vi "Yokogawa Control.vi"(8 "error in (no error)":errorcluster, 9 "Metadata All":T1={"Data Fields"={"operatorName"="", "project"="", "measurementType"="", "sphere"="", "spectrometer"="", "powerSource"="", "analyzer"="", "fixtureType"="", "lampType"="", "sourceType"="", "testOrientation"="", "model"="", "sample"="", "hours"="", "Amp Gain Range"=""}, "Metadata Disable"={"spectrometer"=enum."Disabled and Grayed Out", "sphere"=enum."Disabled and Grayed Out", "analyzer"=enum."Disabled and Grayed Out", "ampGainRange"=enum."Disabled and Grayed Out"}, "Output Path"=path "C:/Users/dhstuart/Dropbox/CLTC/YokogawaPZ4000/Output"}, 10 "Master":refnum<queue>, 11 "VI in":refnum<vi>) -> (0 "error out":errorcluster, 2 "Electrical Data 2":T4)   [LabVIEW 2013]
uses:
  MeasurementControl Message Queue Folder/Message Cluster.ctl
  YokogawaPZ4000/controls/electrical2.ctl
  controls/Metadata all typedef.ctl
  controls/Metadata typedef.ctl
  controls/Metadata disable typedef.ctl
  YokogawaPZ4000/Acquisition/YKPZ400 Acquisition.lvlib
  MeasurementControl Message Queue Folder/MeasurementControl Message Queue.lvlib
  controls/Metadata.lvlib
panel:
  in  "Boolean":bool
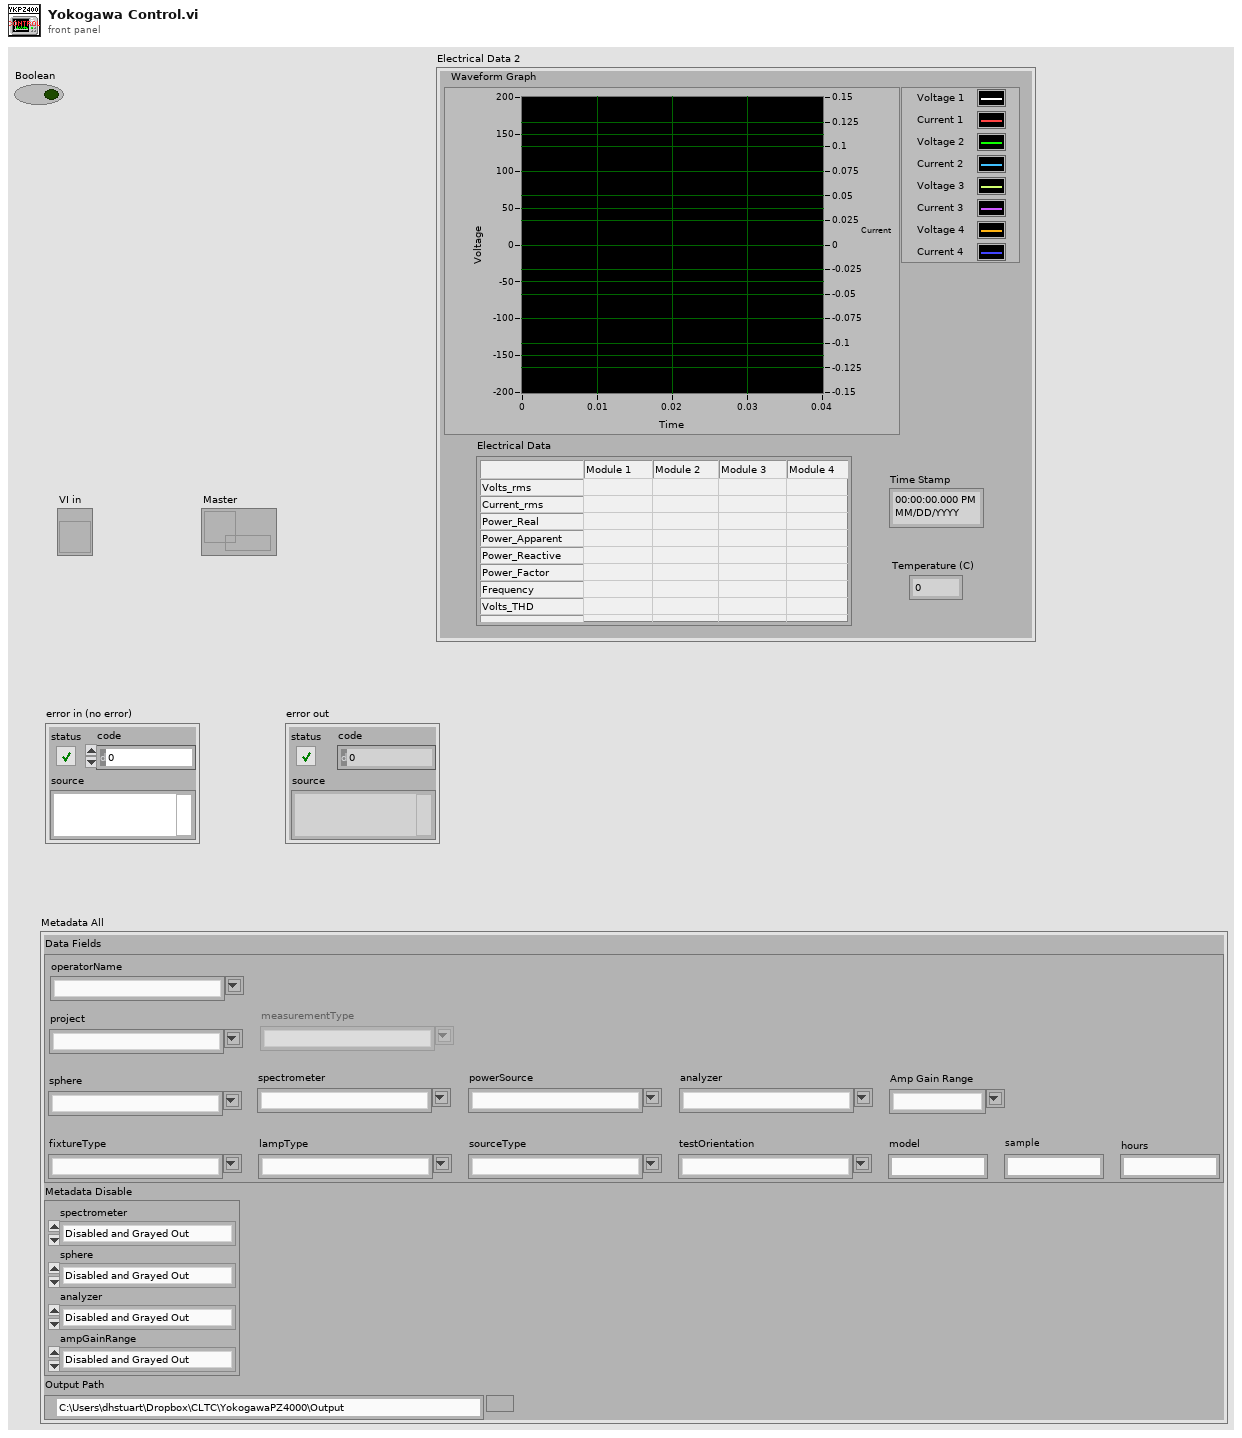
[diagram p1: front panel]
types:
  T1 = typedef "Metadata.lvlib/Metadata all typedef.ctl" = cluster{"Data Fields":T2, "Metadata Disable":T3, "Output Path":path}
  T2 = typedef "Metadata.lvlib/Metadata typedef.ctl" = cluster{"operatorName":string, "project":string, "measurementType":string, "sphere":string, "spectrometer":string, "powerSource":string, "analyzer":string, "fixtureType":string, "lampType":string, "sourceType":string, "testOrientation":string, "model":string, "sample":string, "hours":string, "Amp Gain Range":string}
  T3 = typedef "Metadata.lvlib/Metadata disable typedef.ctl" = cluster{"spectrometer":enum8{"Enabled", "Disabled", "Disabled and Grayed Out"}, "sphere":enum8{"Enabled", "Disabled", "Disabled and Grayed Out"}, "analyzer":enum8{"Enabled", "Disabled", "Disabled and Grayed Out"}, "ampGainRange":enum8{"Enabled", "Disabled", "Disabled and Grayed Out"}}
  T4 = typedef "Yokogawa.lvlib/YKPZ400 Acquisition.lvlib/electrical2.ctl" = cluster{"Time Stamp":timestamp, "Temperature (C)":dbl, "Electrical Data":string[][], "Waveform Graph":waveform(dbl)[]}
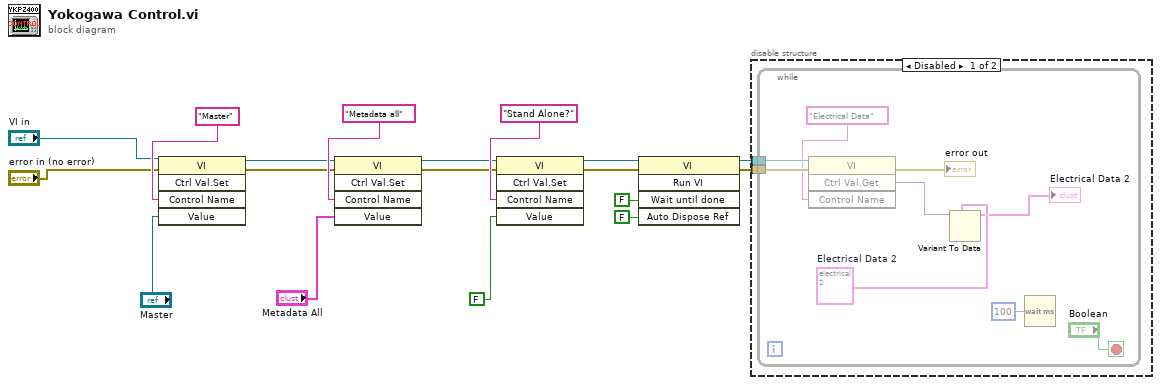
[diagram p0: block diagram]
diagram:
  n1 = invoke class="VI" method="Ctrl Val.Set"(reference="VI in", error in="error in (no error)", "Control Name"="Master", "Value"="Master") -> (reference out=w3:refnum<vi>, error out=w2:errorcluster)  [unwired: 1 in, 3 out]
  n2 = invoke class="VI" method="Ctrl Val.Set"(reference=w3, error in=w2, "Control Name"="Metadata all", "Value"="Metadata All") -> (reference out=w5:refnum<vi>, error out=w4:errorcluster)  [unwired: 1 in, 3 out]
  n3 = invoke class="VI" method="Ctrl Val.Set"(reference=w5, error in=w4, "Control Name"="Stand Alone?", "Value"=FALSE) -> (reference out=w9:refnum<vi>, error out=w8:errorcluster)  [unwired: 1 in, 3 out]
  n4 = invoke class="VI" method="Run VI"(reference=w9, error in=w8, "Wait until done"=FALSE ("Wait Until Done"), "Auto Dispose Ref"=FALSE ("Auto Dispose Reference")) -> (reference out=w18:refnum<vi>, error out=w15:errorcluster)  [unwired: 1 in, 3 out]
  n5 = disable-structure shown="Disabled" {
    disable-tunnel: w18 -> [w20 _]
    disable-tunnel: w15 -> [w19 _]
    frame Disabled {
      n6 = while {
        tunnel: w20 -> [w29]
        tunnel: w19 -> [w28]
        stop <- "Boolean" stop-if-true
        w22 = T4 {"Time Stamp"=timestamp(0 s since 1904-01-01), "Temperature (C)"=0.0, "Electrical Data"=[], "Waveform Graph"=[]}  # Electrical Data 2
        n7 = invoke class="VI" method="Ctrl Val.Get"(reference=w29, error in=w28, "Control Name"="Electrical Data") -> (error out=→"error out":errorcluster, "Get Control Value Variant"=w25:variant)  [unwired: 1 in, 2 out]
        n8 = Variant To Data(type=w22, Variant=w25) -> (data=→"Electrical Data 2":T4)  [unwired: 1 in, 1 out]
        n9 = Wait (ms)(milliseconds to wait=u32 100) -> ()  [unwired: 1 out]
      }
    }
    frame Enabled {
    }
  }
